vi "Filter Event Data.vi"(8 "error in (no error)":errorcluster, 10 "EventFilter Reference":T1, 11 "TreeItemCloseMsg In":refnum<class "TreeItemCloseMsg.lvclass">) -> (0 "error out":errorcluster, 2 "Discard?":bool, 3 "TreeItemCloseMsg Out":refnum<class "TreeItemCloseMsg.lvclass">)   [LabVIEW 2017, in "ActorEvents.lvlib" / "TreeItemCloseMsg.lvclass"]
uses:
  TreeItemCloseMsg.lvclass
  IEventFilter/EventFilter Reference.ctl
  IEventFilter/IEventFilter.lvclass
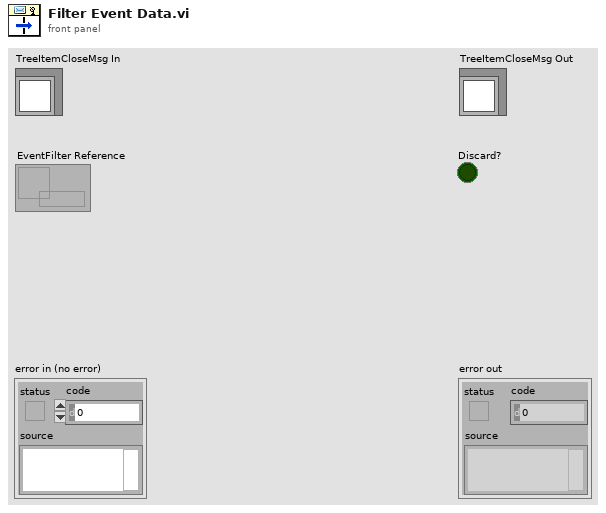
[diagram p1: front panel]
types:
  T1 = typedef "ActorEvents.lvlib/IEventFilter.lvclass/EventFilter Reference.ctl" = refnum<data-value>
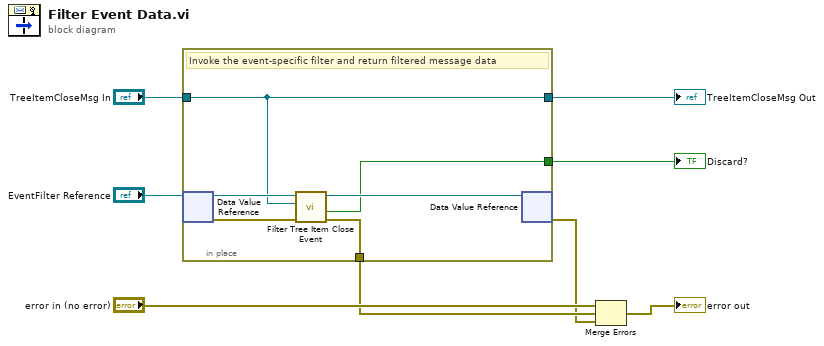
[diagram p0: block diagram]
diagram:
  n1 = in-place {
    in-place-border: "TreeItemCloseMsg In" -> [w9]
    in-place-border: [w9] -> w5
    in-place-border: [w10] -> w3
    in-place-border: [w11] -> w1
    # "Invoke the event-specific filter and return filtered message data"
    n2 = in-place-dvr #1("EventFilter Reference") -> (w14:refnum<class "IEventFilter.lvclass">, w12:errorcluster)
    n3 = call-dynamic "Filter Tree Item Close Event.vi"("error in (no error)"=w12, "TreeItemCloseMsg"=w9, "IEventFilter in"=w14) -> ("error out"=w10:errorcluster, "Discard?"=w11:bool, "IEventFilter out"=w13:refnum<class "IEventFilter.lvclass">)  [unwired: 6 in]
    n4 = in-place-dvr #1(w13) -> (w2:errorcluster)  [unwired: 1 out]
  }
  "TreeItemCloseMsg Out" <- w5
  "Discard?" <- w1
  n5 = Merge Errors("error in (no error)", w3, w2) -> (→"error out":errorcluster)
